vi "CheckFileExist.vi"(8 "error in (no error) 2":errorcluster, 10 "Interactive":bool=TRUE, 11 "File Path":path) -> (0 "error out":errorcluster, 1 "file or folder exists?":bool, 2 "Overwrite":bool, 3 "File out":path)   [LabVIEW 2024]
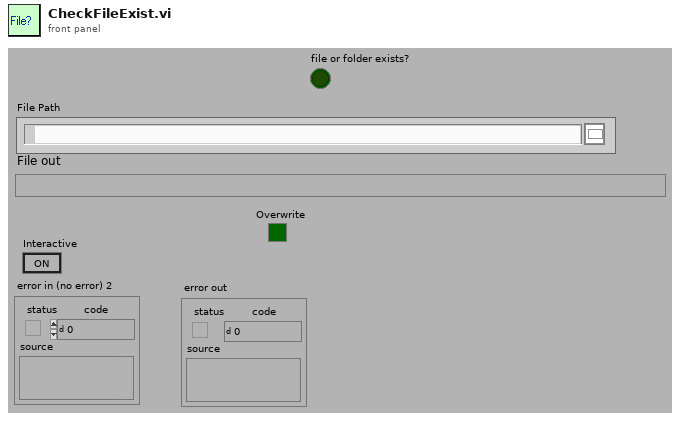
[diagram p1: front panel]
types:
  T1 = enum32{"existing file", "new file", "new or existing file", "existing dir", "new dir", "new or existing dir", "existing file (use LLBs)", "new file (use LLBs)", "new or existing file (use LLBs)", "new or existing file or directory (use LLBs)", "existing dir (use LLBs)", "new dir (use LLBs)", "new or existing dir (use LLBs)", "existing file or dir", "new file or dir", "new or existing file or dir", "existing file or dir (use LLBs)", "new file or dir (use LLBs)"}
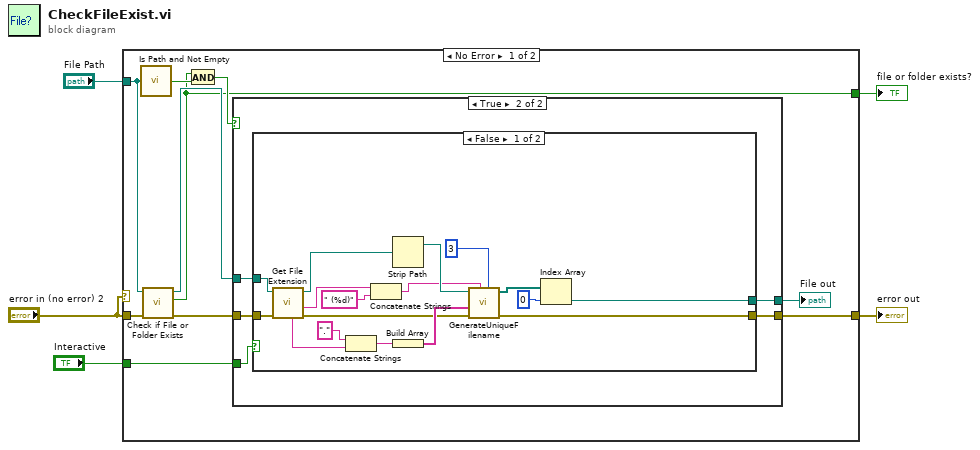
[diagram p0: block diagram]
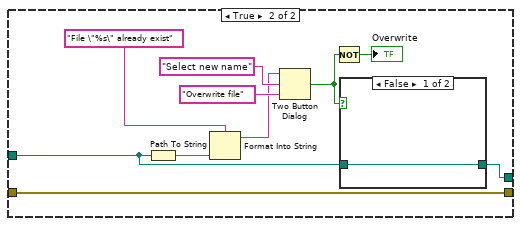
[diagram p3: hidden frame]
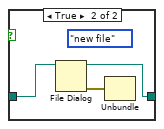
[diagram p4: hidden frame]
diagram:
  n1 = case shown="No Error" "error in (no error) 2" {
    tunnel: "Interactive" -> [w14 _]
    tunnel: [w13 w54] -> w4
    tunnel: "error in (no error) 2" -> [w12 w54]
    tunnel: [w7 _] -> w2
    tunnel: "File Path" -> [w6 _]
    frame No Error {
      n2 = call <vilib>:"Is Path and Not Empty.vi"("path"=w6) -> ("Is Path and Not Empty?"=w9:bool)  [unwired: 4 in]
      n3 = call <vilib>:"Check if File or Folder Exists.vi"("error in (no error)"=w12, "path"=w6) -> ("error out"=w11:errorcluster, "file or folder exists?"=w7:bool, "dup path"=w8:path)  [unwired: 7 in]
      n4 = And(x=w7, y=w9) -> (x .and. y?=w10:bool)
      n5 = case shown="True" w10 {
        tunnel: w8 -> [w17 w21]
        tunnel: [w17 w22] -> w15
        tunnel: w14 -> [_ w20]
        tunnel: w11 -> [w16 w19]
        tunnel: [w16 w18] -> w13
        frame False {
        }
        frame True {
          n6 = case shown="False" w20 {
            tunnel: [w35 w49] -> w22
            tunnel: w21 -> [w33 w45]
            tunnel: w19 -> [w32 w41]
            tunnel: [w39 w41] -> w18
            frame False {
              n7 = call <vilib>:"Get File Extension.vi"("error in (no error)"=w32, "file"=w33) -> ("error out"=w23:errorcluster, "filename without extension"=w31:string, "dup file"=w26:path, "unmodified file extension"=w27:string)  [unwired: 5 in, 1 out]
              n8 = Concatenate Strings("." ("string"), w27) -> (w25:string)
              n9 = Concatenate Strings(w31, " (%d)" ("string")) -> (w29:string)
              n10 = Strip Path(path=w26) -> (stripped path=w34:path)  [unwired: 1 out]
              n11 = Build Array(w25) -> (w37:string[])
              n12 = call "GenerateUniqueFilename.vi"("Index digits"=3, "format string"=w29, "Error In"=w23, "File name suffixes"=w37, "Folder Path Control"=w34) -> ("Error Out"=w39:errorcluster, "Paths"=w38:path[])  [unwired: 5 out]
              n13 = Index Array(array=w38, index=0) -> (element=w35:path)
            }
            frame True {
              n14 = Path To String(path=w45) -> (string=w44:string)
              n15 = Format Into String(format string="File \"%s\" already exist", w44) -> (resulting string=w42:string)  [unwired: 2 in, 1 out]
              n16 = Two Button Dialog(message=w42, 1:"Overwrite file", 2:"Select new name") -> (T button?=w46:bool)
              n17 = Not(x=w46) -> (.not. x?=→"Overwrite":bool)
              n18 = case shown="False" w46 {
                tunnel: [w50 w53] -> w49
                tunnel: w45 -> [w50 w52]
                frame False {
                }
                frame True {
                  (unwired) T1."new file" ("select mode (2)")
                  n19 = File Dialog(11:w52) -> (0:w51:errorcluster, 3:w53:path)  [unwired: 1 in, 7 out]
                  n20 = Unbundle(w51) -> ()  [unwired: 3 out]
                }
              }
            }
          }
        }
      }
      "File out" <- w15
    }
    frame Error {
    }
  }
  "error out" <- w4
  "file or folder exists?" <- w2
